vi "demo.vi"() -> ()   [LabVIEW 2023]
uses:
  <vilib>/numeric/Random Number (Range) DBL.vi
panel:
  out "output":string
  out "Numeric":dbl
  out "body":string
  out "headers":string
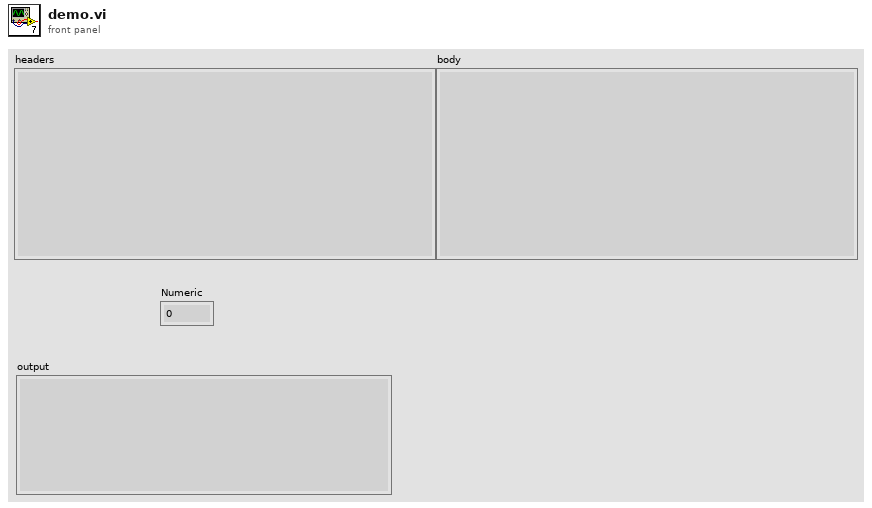
[diagram p1: front panel]
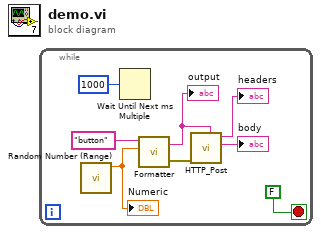
[diagram p0: block diagram]
diagram:
  n1 = while {
    stop <- FALSE stop-if-true
    n2 = call-poly <vilib>:"Random Number (Range).vi"() -> ("number"=w1:dbl)  [unwired: 11 in]
    "Numeric" <- w1
    n3 = Wait Until Next ms Multiple(millisecond multiple=u32 1000) -> ()  [unwired: 1 out]
    n4 = call "Formatter.vi"("Variant"=w1, "ID"="button" ("string")) -> ("error out"=w5:errorcluster, "output"=w4:string)  [unwired: 2 in]
    "output" <- w4
    n5 = call "HTTP_Post.vi"("data"=w4, "error in (no error)"=w5) -> ("body"=→"body":string, "headers"=→"headers":string)  [unwired: 5 in, 1 out]
  }
